vi "Emergency Shutoff.vi"(8 "Error In":errorcluster, 11 "ECU COM Port":refnum<visa-resource-name>) -> (0 "Error Out":errorcluster, 3 "ECU COM Port Out":refnum<visa-resource-name>)   [LabVIEW 2017]
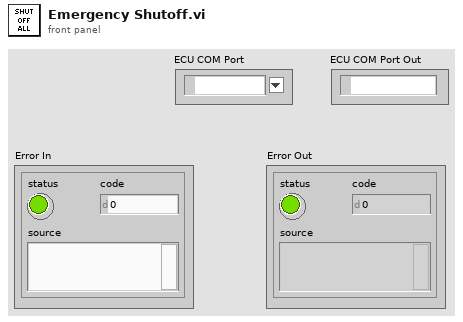
[diagram p1: front panel]
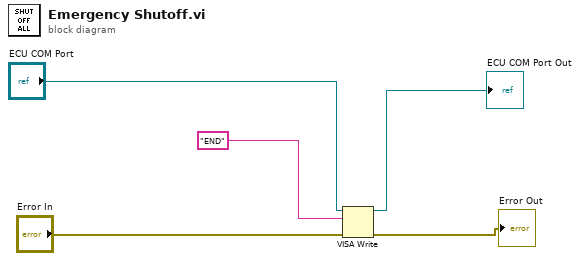
[diagram p0: block diagram]
diagram:
  n1 = VISA Write(VISA resource name="ECU COM Port", write buffer="END", error in (no error)="Error In") -> (VISA resource name out=→"ECU COM Port Out":refnum<visa-resource-name>, error out=→"Error Out":errorcluster)  [unwired: 1 out]
